vi "PCAN_WRITE.vi"(7 "pathCAN_DLL":path, 8 "error in (no error)":errorcluster, 11 "TPCANMsg":T1={"ID"=0, "MSGTYPE"=128, "LEN"=0, "Data"=[]} {"ID" format="%x"; "MSGTYPE" items=["STATUS"=128, "EXTENDED"=2, "RTR"=1, "DATA MSG"=0]}) -> (0 "error out":errorcluster, 3 "error":T2 items=["CAN_ERR_OK"=0, "CAN_ERR_XMTFULL"=1, "CAN_ERR_OVERRUN"=2, "CAN_ERR_BUSLIGHT"=4, "CAN_ERR_BUSHEAVY"=8, "CAN_ERR_BUSOFF"=16, "CAN_ERR_QRCVEMPTY"=32, "CAN_ERR_QOVERRUN"=64, "CAN_ERR_QXMTFULL"=128, "CAN_ERR_REGTEST"=256, "CAN_ERR_NOVXD"=512, "CAN_ERR_HWINUSE"=1024, "CAN_ERR_NETINUSE"=2048, "CAN_ERR_ILLHW"=5120, "CAN_ERR_ILLNET"=6144, "CAN_ERR_ILLCLINET"=7168, "CAN_ERR_RESOURCE"=8192, "CAN_ERR_ILLPARAMTYPE"=16384, "CAN_ERR_ILLPARAMVAL"=32768, "CAN_ERR_UNKNOWN"=65536])   [LabVIEW 2023, in "pCANLib.lvlib"]
doc: "///////////////////////////////////////////////////////////////////////////////\n// CAN_Write()\n// Schreibt eine Message \n// moegliche Fehler: NOVXD RESOURCE BUSOFF QXMTFULL\n//\n\nDWORD __stdcall CAN_Write( TPCANMsg* pMsgBuff);"
uses:
  pCANLib.lvlib
  PCAN_ERROR.ctl
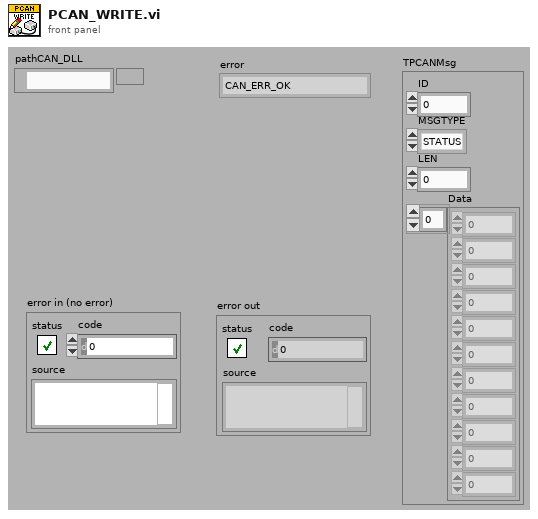
[diagram p1: front panel]
types:
  T1 = cluster{"ID":u32, "MSGTYPE":u8, "LEN":u8, "Data":u8[]}
  T2 = typedef "pCANLib.lvlib/PCAN_ERROR.ctl" = i32
  T3 = enum16{"big-endian, network order", "native, host order", "little-endian"}
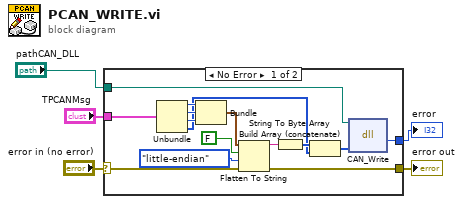
[diagram p0: block diagram]
diagram:
  n1 = case shown="No Error" "error in (no error)" {
    selector: "error in (no error)" -> [w8 w21]
    tunnel: [w20 _] -> w3
    tunnel: [w7 w21] -> w4
    tunnel: "TPCANMsg" -> [w19 _]
    tunnel: "pathCAN_DLL" -> [w6 _]
    frame No Error {
      n2 = Unbundle(w19) -> ("ID"=w18:u32, "MSGTYPE"=w17:u8, "LEN"=w16:u8, "Data"=w12:u8[])
      n3 = Bundle("ID"=w18, "MSGTYPE"=w17, "LEN"=w16) -> (w15:cluster{"ID":u32, "MSGTYPE":u8, "LEN":u8})  [unwired: 1 out]
      n4 = Flatten To String(anything=w15, prepend array or string size? (T)=FALSE, byte order (0:big-endian, network order)=T3."little-endian", error in (no error)=w8) -> (data string=w14:string, error out=w7:errorcluster)  [unwired: 1 out]
      n5 = String To Byte Array(string=w14) -> (unsigned byte array=w13:u8[])
      n6 = Build Array (concatenate)(w13, w12) -> (w11:u8[])
      n7 = dll-call lib="D:/PCAN/PCAN/PCAN Driver/PCAN_Driver/PCAN_USB.DLL" fn="CAN_Write"(path in=w6, "pMsgBuff"=w11) -> ("return type"=w20:i32)  [unwired: 3 in, 2 out]
    }
    frame Error {
    }
  }
  "error out" <- w4
  "error" <- w3
